vi "REM IO - Compare ECAT Vars.vi"(8 "Fehler (Eingang, kein Fehler)":errorcluster, 11 "I/O Vars In":T1[](array[typedef]) {"VS ref" format="%.0x"}) -> (0 "Fehler (Ausgang)":errorcluster, 3 "I/O Vars Out":T1[](array[typedef]) {"VS ref" format="%.0x"})   [LabVIEW 2017, in "Scan Engine Custom Device.lvlib"]
uses:
  Scan Engine Custom Device.lvlib
  Type Defs/REM IO ECAT Slave IOV Cluster.ctl
  <vilib>/NI Veristand/Custom Device API/Custom Device Item Ref.ctl
  Type Defs/UDV Data Type.ctl
  Globals/Property Strings.vi
  <vilib>/NI Veristand/Custom Device API/Get Item Property (String).vi
  <vilib>/NI Veristand/Custom Device API/Get Item Property (I32).vi
  Globals/Error Strings.vi
  <vilib>/NI VeriStand/Custom Device API/Custom Device API.lvlib
  <vilib>/NI Veristand/Custom Device Tools/Custom Device Utility Library/Custom Device Utility Library.lvlib
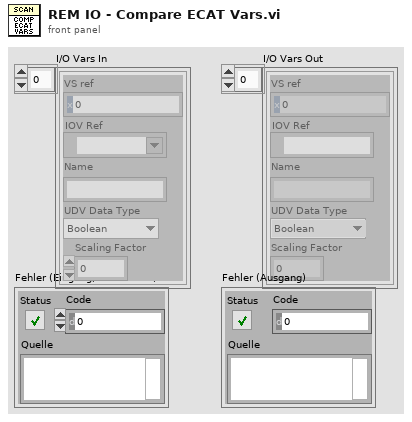
[diagram p1: front panel]
types:
  T1 = typedef "Scan Engine Custom Device.lvlib/REM IO ECAT Slave IOV Cluster.ctl" = cluster{"VS ref":T2, "IOV Ref":refnum<k21>, "Name":string, "UDV Data Type":T3, "Scaling Factor":dbl}
  T2 = typedef "Custom Device API.lvlib/Custom Device Item Ref.ctl" = u64
  T3 = typedef "Scan Engine Custom Device.lvlib/UDV Data Type.ctl" = enum16{"Boolean", "Fixed Point", "Int8", "Int16", "Int32", "Int64", "U32 Bit Field", "UInt8", "UInt16", "UInt32", "UInt64", "Other"}
  T4 = typedef "Custom Device API.lvlib/Custom Device Item Info.ctl" = cluster{"Name":string, "Is Channel":bool, "GUID":string, "Is Waveform":bool}
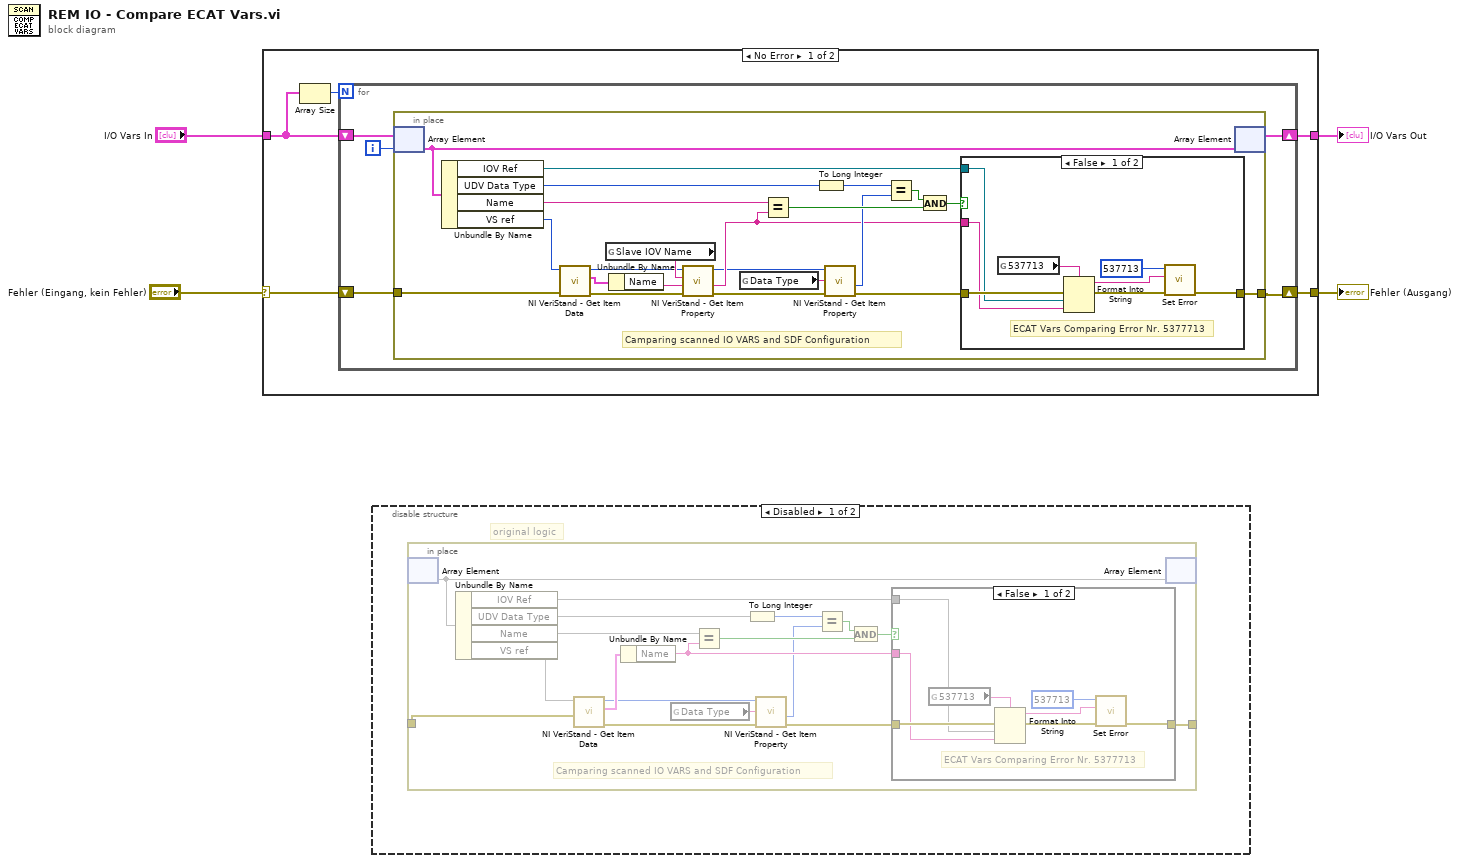
[diagram p0: block diagram]
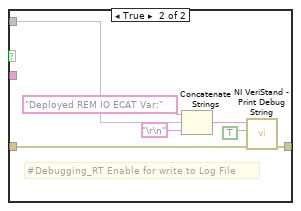
[diagram p2: hidden frame]
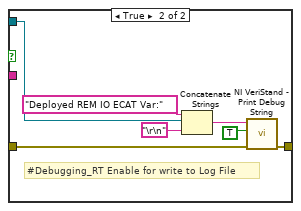
[diagram p4: hidden frame]
diagram:
  n1 = case shown="No Error" "Fehler (Eingang, kein Fehler)" {
    selector: "Fehler (Eingang, kein Fehler)" -> [w8 w53]
    tunnel: [w5 w52] -> w1
    tunnel: [w7 w53] -> w4
    tunnel: "I/O Vars In" -> [w6 w52]
    frame No Error {
      n2 = Array Size(array=w6) -> (size(s)=w9:i32)
      n3 = for {
        N: w9 -> [_]
        shift-right: [w12] -> w7
        shift-left: w8 -> [w13]
        shift-right: [w10] -> w5
        shift-left: w6 -> [w11]
        i -> [w14]
        n4 = in-place {
          in-place-border: w13 -> [w34]
          in-place-border: [w29] -> w12
          # "Camparing scanned IO VARS and SDF Configuration"
          n5 = in-place-array #1(w11, w14) -> (w25:T1)
          n6 = Unbundle By Name(w25) -> ("IOV Ref"=w27:refnum<k21>, "UDV Data Type"=w28:T3, "Name"=w24:string, "VS ref"=w26:T2)
          n7 = call <vilib>:"NI VeriStand - Get Item Data.vi"("error in (no error)"=w34, "Item Ref in"=w26) -> ("error out"=w19:errorcluster, "Item Info"=w36:T4, "Item Ref out"=w16:T2)  [unwired: 6 in, 1 out]
          n8 = global read "Property Strings.vi" "Slave IOV Name"() -> (w21:string)
          n9 = Unbundle By Name(w36) -> ("Name"=w20:string)
          n10 = call-poly <vilib>:"NI VeriStand - Get Item Property.vi"("error in (no error)"=w19, "Default Value"=w20, "Property Name"=w21, "Item Ref in"=w16) -> ("error out"=w18:errorcluster, "Value"=w17:string, "Item Ref out"=w15:T2)  [unwired: 4 in, 1 out]
          n11 = global read "Property Strings.vi" "Data Type"() -> (w35:string)
          n12 = Equal?(x=w24, y=w17) -> (x = y?=w32:bool)
          n13 = To Long Integer(number=w28) -> (32bit integer=w22:i32)
          n14 = call-poly <vilib>:"NI VeriStand - Get Item Property.vi"("error in (no error)"=w18, "Property Name"=w35, "Item Ref in"=w15) -> ("error out"=w30:errorcluster, "Value"=w23:i32)  [unwired: 5 in, 2 out]
          n15 = Equal?(x=w22, y=w23) -> (x = y?=w33:bool)
          n16 = And(x=w33, y=w32) -> (x .and. y?=w31:bool)
          n17 = case shown="False" w31 {
            tunnel: w30 -> [w40 w51]
            tunnel: [w39 w50] -> w29
            tunnel: w27 -> [w38 w46]
            tunnel: w17 -> [w37 _]
            frame False {
              # "ECAT Vars Comparing Error Nr. 5377713"
              n18 = global read "Error Strings.vi" "537713"() -> (w41:string)
              n19 = Format Into String(format string=w41, error in=w40, w38, w37) -> (resulting string=w43:string, error out=w42:errorcluster)  [unwired: 1 in]
              n20 = call "Set Error.vi"("error in (no error)"=w42, "Message"=w43, "Code"=537713 ("error code (0)")) -> ("error out"=w39:errorcluster)  [unwired: 8 in]
            }
            frame True {
              # "#Debugging_RT Enable for write to Log File"
              n21 = Concatenate Strings("Deployed REM IO ECAT Var:", w46, "\r\n") -> (w49:string)
              n22 = call <vilib>:"NI VeriStand - Print Debug String.vi"("error in (no error)"=w51, "Add to log file? (T)"=TRUE, "Message"=w49) -> ("error out"=w50:errorcluster)  [unwired: 8 in]
            }
          }
          n23 = in-place-array #1(w25) -> (w10:T1[])  [unwired: 1 out]
        }
      }
    }
    frame Error {
    }
  }
  "I/O Vars Out" <- w1
  "Fehler (Ausgang)" <- w4
  n24 = disable-structure shown="Disabled" {
    frame Disabled {
      # "original logic"
      n25 = in-place {
        in-place-border: _ -> [w67]
        in-place-border: [w62] -> _
        # "Camparing scanned IO VARS and SDF Configuration"
        n26 = in-place-array #2() -> (w57)  [unwired: 2 in]
        n27 = Unbundle By Name(w57) -> ("IOV Ref"=w60, "UDV Data Type"=w61, "Name"=w56, "VS ref"=w58)
        n28 = call <vilib>:"NI VeriStand - Get Item Data.vi"("error in (no error)"=w67, "Item Ref in"=w58) -> ("error out"=w70:errorcluster, "Item Info"=w71:T4, "Item Ref out"=w69:T2)  [unwired: 6 in, 1 out]
        n29 = Unbundle By Name(w71) -> ("Name"=w59:string)
        n30 = global read "Property Strings.vi" "Data Type"() -> (w68:string)
        n31 = Equal?(x=w56, y=w59) -> (x = y?=w65:bool)
        n32 = To Long Integer(number=w61) -> (32bit integer=w54:i32)
        n33 = call-poly <vilib>:"NI VeriStand - Get Item Property.vi"("error in (no error)"=w70, "Property Name"=w68, "Item Ref in"=w69) -> ("error out"=w63:errorcluster, "Value"=w55:i32)  [unwired: 5 in, 2 out]
        n34 = Equal?(x=w54, y=w55) -> (x = y?=w66:bool)
        n35 = And(x=w66, y=w65) -> (x .and. y?=w64:bool)
        n36 = case shown="False" w64 {
          tunnel: w63 -> [w75 w86]
          tunnel: [w74 w85] -> w62
          tunnel: w60 -> [w73 w81]
          tunnel: w59 -> [w72 _]
          frame False {
            # "ECAT Vars Comparing Error Nr. 5377713"
            n37 = global read "Error Strings.vi" "537713"() -> (w76:string)
            n38 = Format Into String(format string=w76, error in=w75, w73, w72) -> (resulting string=w78:string, error out=w77:errorcluster)  [unwired: 1 in]
            n39 = call "Set Error.vi"("error in (no error)"=w77, "Message"=w78, "Code"=537713 ("error code (0)")) -> ("error out"=w74:errorcluster)  [unwired: 8 in]
          }
          frame True {
            # "#Debugging_RT Enable for write to Log File"
            n40 = Concatenate Strings("Deployed REM IO ECAT Var:", w81, "\r\n") -> (w84:string)
            n41 = call <vilib>:"NI VeriStand - Print Debug String.vi"("error in (no error)"=w86, "Add to log file? (T)"=TRUE, "Message"=w84) -> ("error out"=w85:errorcluster)  [unwired: 8 in]
          }
        }
        n42 = in-place-array #2(w57) -> ()  [unwired: 2 out]
      }
    }
    frame Enabled {
    }
  }
